vi "Inst.KH7008.getChannel.vi"(6 "channel":T1=1 min=1 max=8 step=1, 8 "error in (no error)":errorcluster, 11 "Inst.Krohn-Hite-7008 in":refnum<class "Inst.Krohn-Hite-7008.lvclass">) -> (0 "error out":errorcluster, 2 "channelProperties":T2={"channel"=1, "gain"=enum."10", "input"=enum."SE+", "shunt"=enum."50", "couple"=enum."DC", "filter"=enum."ON"} {"channel" min=1 max=8 step=1}, 3 "Inst.Krohn-Hite-7008 out":refnum<class "Inst.Krohn-Hite-7008.lvclass">)   [LabVIEW 2019, in "Inst.KH7008.lvlib" / "Inst.Krohn-Hite-7008.lvclass"]
uses:
  Inst.Krohn-Hite-7008.lvclass
  KH7008/typedefs/channel--numeric.ctl
  KH7008/KH7008.lvlib
  KH7008/typedefs/gain--enum.ctl
  KH7008/typedefs/Input--Enum.ctl
  KH7008/typedefs/shunt--enum.ctl
  KH7008/typedefs/couple--Enum.ctl
  KH7008/typedefs/Filter--Enum.ctl
  KH7008/typedefs/channelProperties--Cluster.ctl
  KH7008/typedefs/allChannelProperties--Array.ctl
  Typedefs/getAllChannelsResponse--Cluster.ctl
  1fdc1f3d-332e-4594-8a59-3c61ed5849a6.vi
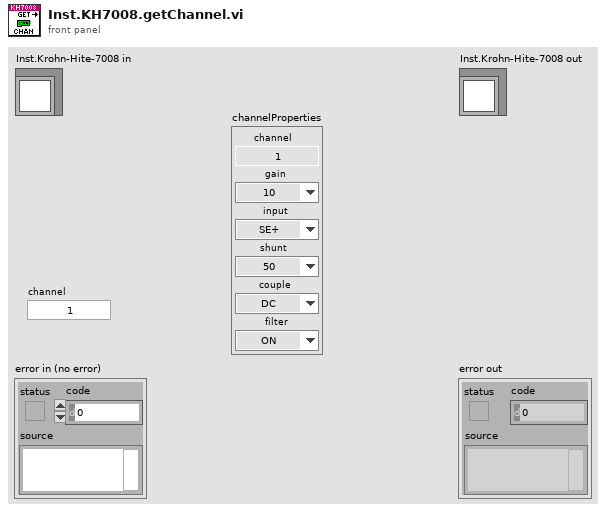
[diagram p1: front panel]
types:
  T1 = typedef "KH7008.lvlib/channel--numeric.ctl" = u16
  T2 = typedef "KH7008.lvlib/channelProperties--Cluster.ctl" = cluster{"channel":T1, "gain":T3, "input":T4, "shunt":T5, "couple":T6, "filter":T7}
  T3 = typedef "KH7008.lvlib/gain--enum.ctl" = enum16{"1", "10", "100", "1000"}
  T4 = typedef "KH7008.lvlib/input--enum.ctl" = enum16{"OFF", "SE+", "SE-", "DIFF"}
  T5 = typedef "KH7008.lvlib/shunt--enum.ctl" = enum16{"Open", "50", "500", "5k", "50k", "10M"}
  T6 = typedef "KH7008.lvlib/couple--enum.ctl" = enum16{"AC", "DC"}
  T7 = typedef "KH7008.lvlib/filter--enum.ctl" = enum16{"OFF", "ON"}
  T8 = typedef "Inst.KH7008.lvlib/Inst.Krohn-Hite-7008.lvclass/getAllChannelsResponse--Cluster.ctl" = cluster{"allChannelProperties":T9}
  T9 = typedef "KH7008.lvlib/allChannelProperties--Array.ctl" = T2[]
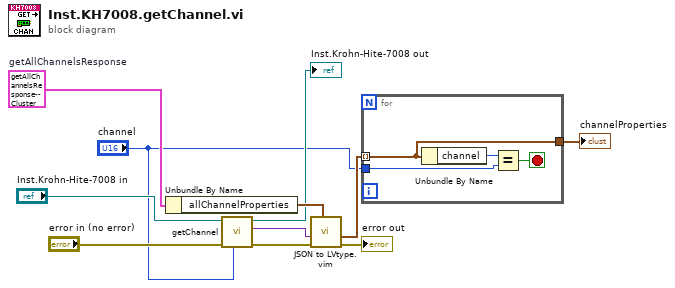
[diagram p0: block diagram]
diagram:
  w11 = T8 {"allChannelProperties"=[{"channel"=1, "gain"=enum."10", "input"=enum."OFF", "shunt"=enum."10M", "couple"=enum."AC", "filter"=enum."OFF"}, {"channel"=2, "gain"=enum."10", "input"=enum."OFF", "shunt"=enum."10M", "couple"=enum."AC", "filter"=enum."OFF"}, {"channel"=3, "gain"=enum."10", "input"=enum."OFF", "shunt"=enum."10M", "couple"=enum."AC", "filter"=enum."OFF"}, {"channel"=4, "gain"=enum."10", "input"=enum."OFF", "shunt"=enum."10M", "couple"=enum."AC", "filter"=enum."OFF"}, {"channel"=5, "gain"=enum."10", "input"=enum."OFF", "shunt"=enum."10M", "couple"=enum."AC", "filter"=enum."OFF"}, {"channel"=6, "gain"=enum."10", "input"=enum."OFF", "shunt"=enum."10M", "couple"=enum."AC", "filter"=enum."OFF"}, {"channel"=7, "gain"=enum."10", "input"=enum."OFF", "shunt"=enum."10M", "couple"=enum."AC", "filter"=enum."OFF"}, {"channel"=7, "gain"=enum."10", "input"=enum."OFF", "shunt"=enum."10M", "couple"=enum."AC", "filter"=enum."OFF"}]}  # getAllChannelsResponse
  n1 = Unbundle By Name(w11) -> ("allChannelProperties"=w8:T9)
  n2 = call-dynamic "getChannel.vi"("channel"="channel", "error in (no error)"="error in (no error)", "Inst.Krohn-Hite-7008 in"="Inst.Krohn-Hite-7008 in") -> ("error out"=w4:errorcluster, "channelProperties"=w3:variant, "Inst.Krohn-Hite-7008 out"=→"Inst.Krohn-Hite-7008 out":refnum<class "Inst.Krohn-Hite-7008.lvclass">)  [unwired: 6 in]
  n3 = call "JSON to LVtype.vim"("type"=w8, "error in (no error)"=w4, "JSON Data in"=w3) -> ("error out"=→"error out":errorcluster, "Data out"=w7:T2[])  [unwired: 7 in]
  n4 = for {
    tunnel: w7 -> [w12] mode=indexing
    tunnel: "channel" -> [w15]
    tunnel: [w12] -> w10
    stop <- w14 stop-if-true
    n5 = Unbundle By Name(w12) -> ("channel"=w13:T1)
    n6 = Equal?(x=w13, y=w15) -> (x = y?=w14:bool)
  }
  "channelProperties" <- w10
